vi "TDR.vi"() -> ()   [LabVIEW 2018]
doc: "PNA-X Example."
uses:
  PNA-X.lvlib
panel:
  out "VISA OUT":refnum<visa-resource-name>
  out "error out":errorcluster
  in  "error in (no error)":errorcluster
  in  "VISA IN":refnum<visa-resource-name>
  out "XY Graph":cluster{"X-Axis":dbl[], "Data":dbl[]}(graph)
  # "1. Select Instrument Source from the \"VISA IN\" drop down.\n2. Run vi"
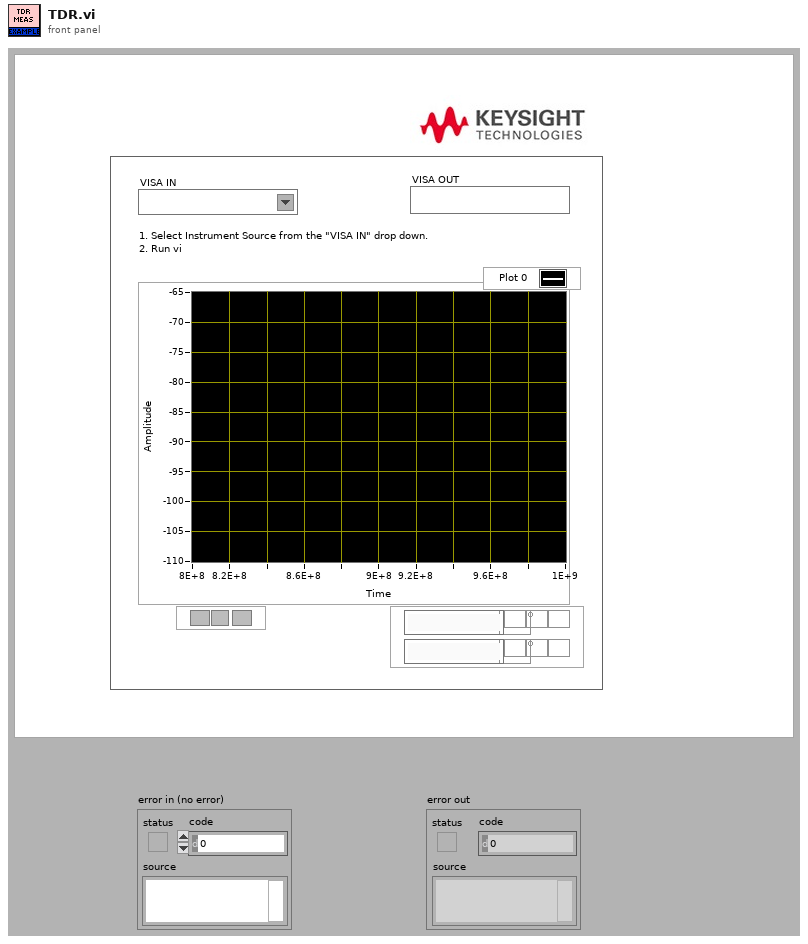
[diagram p1: front panel]
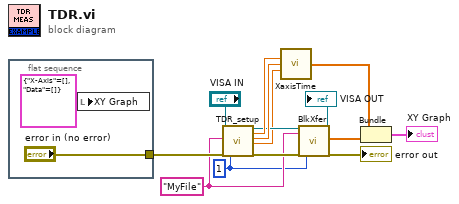
[diagram p0: block diagram]
diagram:
  w4 = 1 ("Channel")
  w5 = "MyFile" ("FileName")
  n1 = flat-sequence {
    tunnel: ["error in (no error)"] -> w9
    frame #0 {
      n2 = local write "XY Graph"(cluster{"X-Axis":dbl[], "Data":dbl[]} {"X-Axis"=[], "Data"=[]} ("XY Graph")) -> ()
    }
  }
  n3 = call "TDR_setup.vi"("VISA IN"="VISA IN", "FileName"=w5, "error in"=w9, "Channel"=w4) -> ("dup VISA session"=w6:refnum<visa-resource-name>, "StartT"=w14:dbl, "StopT"=w13:dbl, "Num Pts"=w1:dbl, "error out"=w7:errorcluster)  [unwired: 11 in]
  n4 = call "XaxisTime.vi"("Start Time"=w14, "Stop Time"=w13, "Points"=w1) -> ("X-Axis"=w12:dbl[])  [unwired: 12 in]
  n5 = call "BlkXfer.vi"("VISA IN"=w6, "FileName"=w5, "error in"=w7, "Channel"=w4) -> ("VISA Out"=→"VISA OUT":refnum<visa-resource-name>, "Data"=w11:dbl[], "error out"=→"error out":errorcluster)  [unwired: 13 in]
  n6 = Bundle("X-Axis"=w12, "Data"=w11) -> (→"XY Graph":cluster{"X-Axis":dbl[], "Data":dbl[]})  [unwired: 1 in]
